vi "KHETS - About.vi"() -> ()   [LabVIEW 2018]
panel:
  out "Additional Information":string
  in  "OK Button":bool
  # "Keithley Hall Effect Test Suite"
  # "Version: 2.0.0             Date: 7/14/2017"
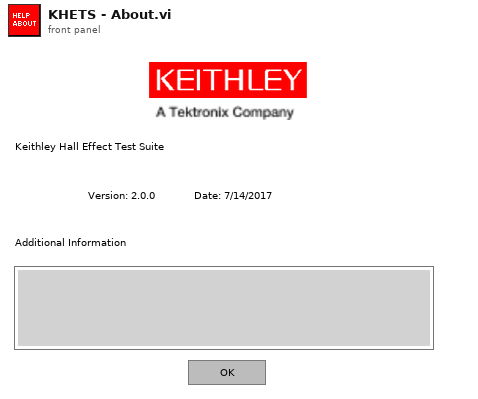
[diagram p1: front panel]
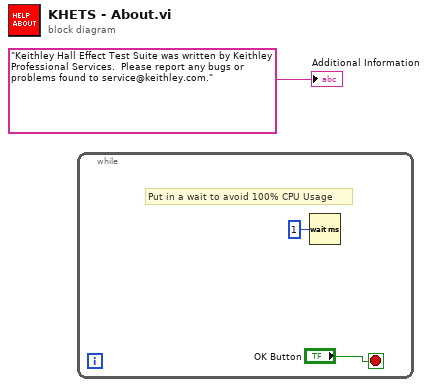
[diagram p0: block diagram]
diagram:
  n1 = while {
    stop <- "OK Button" stop-if-true
    # "Put in a wait to avoid 100% CPU Usage"
    n2 = Wait (ms)(milliseconds to wait=u32 1) -> ()  [unwired: 1 out]
  }
  "Additional Information" <- "Keithley Hall Effect Test Suite was written by Keithley Professional Services.  Please report any bugs or problems found to service@keithley.com." ("Additional Information")
